vi "Pid_v12.vi"() -> ()   [LabVIEW 2020]
panel:
  out "U - Comanda":dbl(graph)=48.656716417098906
  out "Inte":dbl=54.73880596921972
  out "Y - Iesirea":dbl(slide)=48.65671641792066 scale=40.0..60.0
  in  "stop":bool
  out "Deriv":dbl=1.6470380614919122e-10
  out "Y":dbl=48.65671641792066
  out "U- Comanda":dbl(slide)=48.65671641709671 scale=40.0..60.0
  out "u,y,r":cluster{"r-Set point":dbl, dbl, dbl}(graph)={"r-Set point"=48.656716417910445, 48.65671641792066, 48.656716417098906}
  in  "Kd":dbl(slide)=0.1111111111111111 scale=0.0..0.5
  in  "Kp":dbl(slide)=0.3508771929824561 scale=0.0..2.5
  in  "Ki":dbl(slide)=0.8888888888888888 scale=0.0..2.0
  in  "r":dbl(slide)=48.656716417910445 scale=40.0..60.0
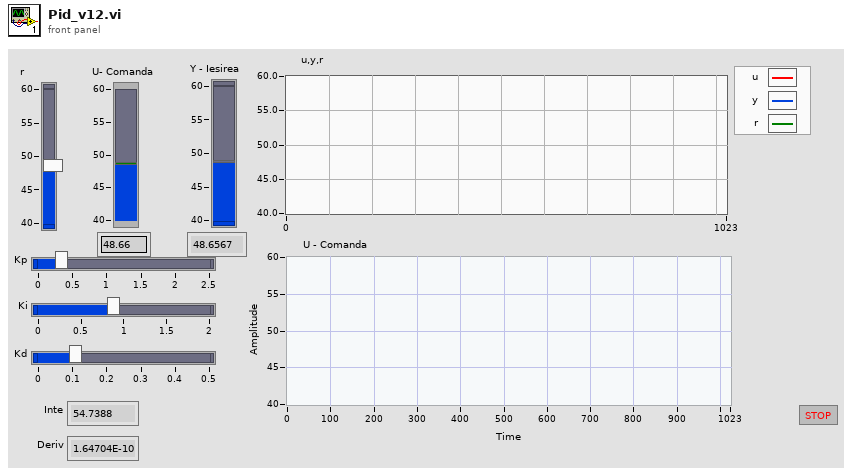
[diagram p1: front panel]
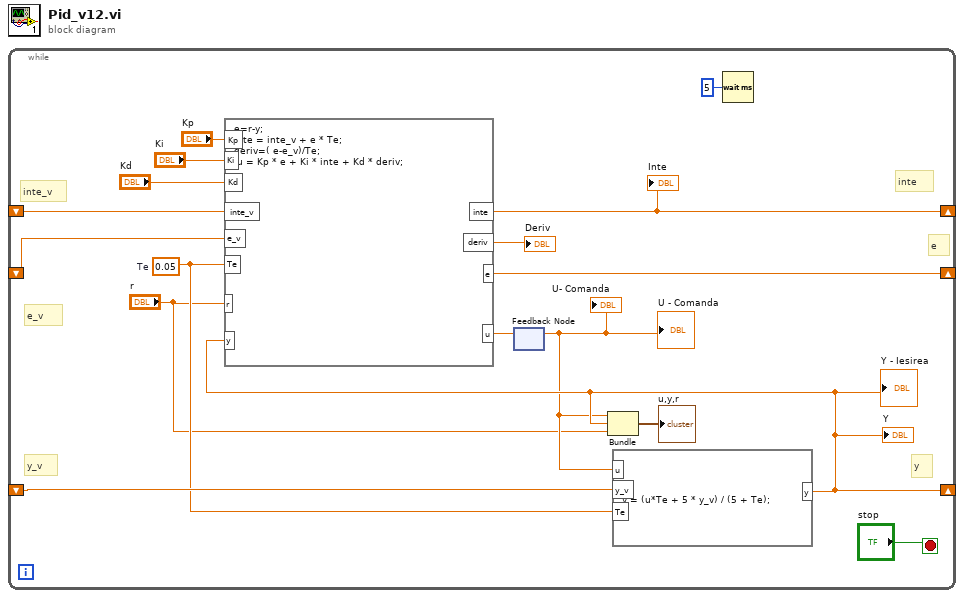
[diagram p0: block diagram]
diagram:
  n1 = while {
    shift-right: [w6] -> _
    shift-left: _ -> [w12]
    shift-right: [w3] -> _
    shift-left: _ -> [w5]
    shift-right: [w13] -> _
    shift-left: _ -> [w14]
    stop <- "stop" stop-if-true
    w4 = 0.05  # Te
    # "e_v"
    # "e"
    # "inte_v"
    # "inte"
    # "y_v"
    # "y"
    n2 = feedback #1() -> (w2:dbl)  [unwired: 1 in]
    "U- Comanda" <- w2
    "U - Comanda" <- w2
    n3 = formula code="y = (u*Te + 5 * y_v) / (5 + Te);"("y_v"=w5, "u"=w2, "Te"=w4) -> ("y"=w3:dbl)
    "Y" <- w3
    "Y - Iesirea" <- w3
    n4 = formula code="e=r-y;\ninte = inte_v + e * Te;\nderiv=( e-e_v)/Te;\n u = Kp * e + Ki * inte + Kd * deriv;"("inte_v"=w14, "Te"=w4, "e_v"=w12, "Kp"="Kp", "Ki"="Ki", "Kd"="Kd", "r"="r", "y"=w3) -> ("inte"=w13:dbl, "deriv"=→"Deriv":dbl, "u"=w7:dbl, "e"=w6:dbl)
    "Inte" <- w13
    n5 = feedback-in #1(w7) -> ()
    n6 = Bundle("u"=w2, "y"=w3, "r"="r") -> (→"u,y,r":cluster{"u":dbl, "y":dbl, "r":dbl})  [unwired: 1 in]
    n7 = Wait (ms)(milliseconds to wait=u32 5) -> ()  [unwired: 1 out]
  }
